vi "Write.vi"(6 "high priority? (F)":bool, 8 "abort (F)":bool, 9 "last element? (F)":bool, 10 "element":cluster{"cmd":string, "data":variant}, 11 "element valid? (T)":bool=TRUE) -> (0 "done?":bool, 2 "channel out":T1)   [LabVIEW 2019, in "Cmd-Data Event Messenger.lvlib"]
doc: "<p>Writes a value to an Event Messenger <a href=\"nihelplauncher://docs/csh?context=lvcore_lvconcepts_channel_wires_intro\">channel</a> so that the value can be read by one or more <a href=\"nihelplauncher://docs/csh?context=lvcore_glang_event_structure\">Event structures</a>. This endpoint waits if the channel is full.</p>"
uses:
  Cmd-Data Event Messenger.lvlib
  <vilib>/event_ctls.llb/usereventprio.ctl
  <resource>/ChannelSupport/_ChannelSupport/GetErrors/FpgaChannelWireNotSupported.xnode
  ChannelOp.ctl
  ))Channel.ctl
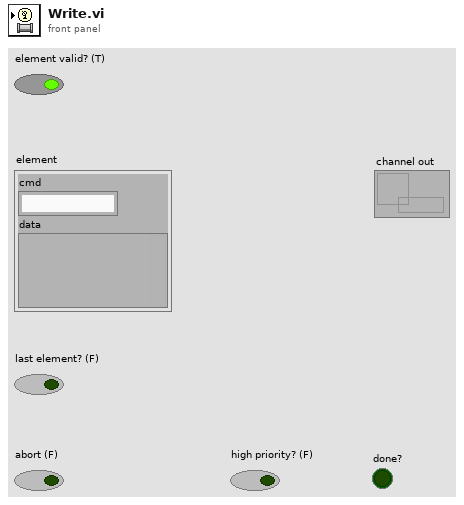
[diagram p1: front panel]
types:
  T1 = typedef "Cmd-Data Event Messenger.lvlib/))Channel.ctl" = refnum<queue>
  T2 = typedef "usereventprio.ctl" = enum32{"high priority", "normal priority"}
  T3 = typedef "Cmd-Data Event Messenger.lvlib/ChannelOp.ctl" = enum16{"init", "write", "register", "replicate", "probe"}
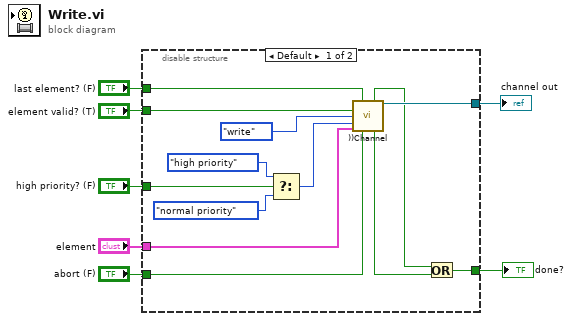
[diagram p0: block diagram]
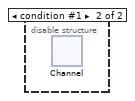
[diagram p2: hidden frame]
diagram:
  n1 = disable-structure shown="Default" {
    disable-tunnel: [w19 _] -> w1
    disable-tunnel: "element" -> [w18 _]
    disable-tunnel: "element valid? (T)" -> [w17 _]
    disable-tunnel: "abort (F)" -> [w16 _]
    disable-tunnel: "last element? (F)" -> [w15 _]
    disable-tunnel: [w12 _] -> w3
    disable-tunnel: "high priority? (F)" -> [w11 _]
    frame condition #0 (active) {
      n2 = Select(t=usereventprio."high priority" ("event priority (normal)"), s=w11, f=usereventprio."normal priority" ("event priority (normal)")) -> (s? t:f=w8:T2)
      n3 = call "))Channel.vi"("last element in"=w15, "valid"=w17, "channelOp"=ChannelOp."write", "event priority (norm)"=w8, "element in"=w18, "abort in"=w16) -> ("last element out"=w14:bool, "channel out"=w19:T1, "aborted?"=w13:bool)  [unwired: 5 in, 2 out]
      n4 = Or(x=w14, y=w13) -> (x .or. y?=w12:bool)
    }
    frame condition #1 {
      n5 = xnode "Channel"() -> ()
    }
  }
  "done?" <- w3
  "channel out" <- w1
